vi "Config Aout Source.vi"(8 "error in":errorcluster, 9 "Loss (Deviation)":u16(ring)=2 items=["Ground", "Bias", "Deviation"], 10 "Capacitance (Deviation)":u16(ring)=2 items=["Ground", "Bias", "Deviation"], 11 "VISA resource name":refnum<visa-resource-name>) -> (0 "error out":errorcluster, 3 "VISA resource name out":refnum<visa-resource-name>)   [LabVIEW 2017, in "Andeen-Hagerling 2700.lvlib"]
doc: "Each of the capacitance and loss analog outputs on the rear panel can be fed from any one of three internal sources; the deviation subsystem, the bias voltage source, or the zero voltage source. This VI selects which among these three sources is connected to each of the rear panel analog outputs."
uses:
  Andeen-Hagerling 2700.lvlib
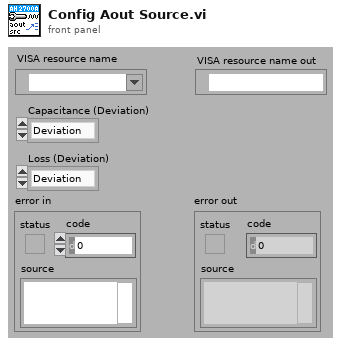
[diagram p1: front panel]
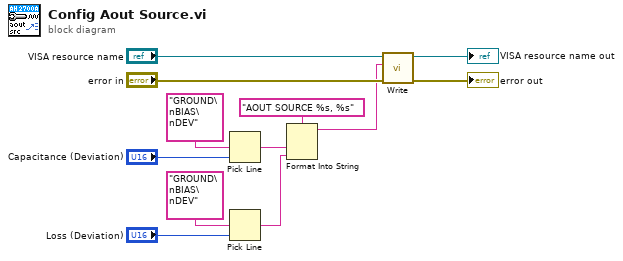
[diagram p0: block diagram]
diagram:
  n1 = Pick Line(multi-line string="GROUND\nBIAS\nDEV", line index="Capacitance (Deviation)") -> (output string=w7:string)  [unwired: 1 in]
  n2 = Pick Line(multi-line string="GROUND\nBIAS\nDEV", line index="Loss (Deviation)") -> (output string=w6:string)  [unwired: 1 in]
  n3 = Format Into String(format string="AOUT SOURCE %s, %s", w7, w6) -> (resulting string=w1:string)  [unwired: 2 in, 1 out]
  n4 = call "Write.vi"("error in"="error in", "command"=w1, "VISA resource name"="VISA resource name") -> ("error out"=→"error out":errorcluster, "VISA resource name out"=→"VISA resource name out":refnum<visa-resource-name>)  [unwired: 7 in]
